vi "Image Dual Threshold [U16].vi"(8 "error in (no error)":errorcluster, 9 "Range":cluster{"Lower value":sgl, "Upper value":sgl}={"Lower value"=128.0, "Upper value"=255.0} {"Upper value" format="%.2f"; "Lower value" format="%.2f"}, 11 "Image in":T1) -> (0 "error out":errorcluster, 1 "CPU (s)":dbl, 3 "Image Out":T1)   [LabVIEW 2021, in "Image.lvlib"]
uses:
  <vilib>/vision/Image Controls.llb/IMAQ Image.ctl
  <vilib>/vision/EDVR.llb/IMAQ ImageToEDVR 2D U16.vi
  Image.lvlib
  Time/Time.lvlib
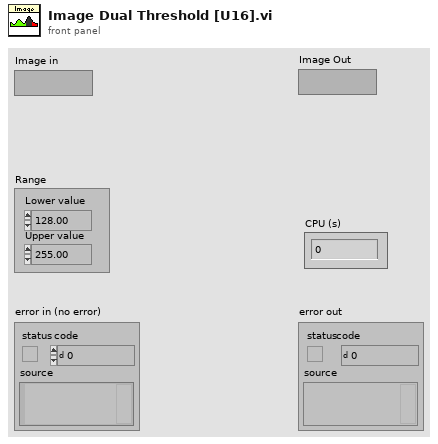
[diagram p1: front panel]
types:
  T1 = typedef "IMAQ Image.ctl" = refnum<image>
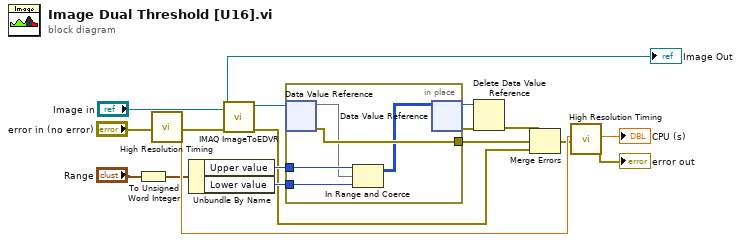
[diagram p0: block diagram]
diagram:
  n1 = To Unsigned Word Integer(number="Range") -> (unsigned 16bit integer=w3:cluster{"Lower value":u16, "Upper value":u16})
  n2 = call "High Resolution Timing.vi"("Error In"="error in (no error)") -> ("elapsed (relative) seconds"=w8:dbl, "Error Out"=w10:errorcluster)  [unwired: 16 in, 1 out]
  n3 = Unbundle By Name(w3) -> ("Upper value"=w15:u16, "Lower value"=w14:u16)
  n4 = call-poly <vilib>:"IMAQ ImageToEDVR.vi"("error out"=w10, "Image"="Image in") -> ("error out"=w4:errorcluster, "EDVR 2D U16"=w17:refnum<data-value>)  [unwired: 7 in, 1 out]
  n5 = in-place {
    in-place-border: w15 -> [w22]
    in-place-border: w14 -> [w21]
    in-place-border: [w20] -> w6
    n6 = in-place-dvr #1(w17) -> (w19:u16[][], w20:errorcluster)
    n7 = In Range and Coerce(upper limit=w22, x=w19, lower limit=w21) -> (coerced(x)=w18:u16[][])  [unwired: 1 out]
    n8 = in-place-dvr #1(w18) -> (w13:refnum<data-value>, w12:errorcluster)
  }
  n9 = Delete Data Value Reference(data value reference=w13, error in=w12) -> (error out=w5:errorcluster)  [unwired: 1 out]
  n10 = Merge Errors(w5, w6, w4) -> (w1:errorcluster)
  n11 = call "High Resolution Timing.vi"("relative seconds (NaN)"=w8, "Error In"=w1) -> ("elapsed (relative) seconds"=→"CPU (s)":dbl, "Error Out"=→"error out":errorcluster)  [unwired: 15 in, 1 out]
  "Image Out" <- "Image in"
